vi "Compose email message.vi"(8 "error in (no error)":errorcluster, 11 "DesignRequest":T1={"Project Folder"=path "D:/inetpub/wwwroot/Designs/341406569189", "Method Name"="EtFlocSedFi", "Inputs"=[{"Label.Text"="UI.Name", "Control Type"=4, "Numeric"=0.0, "Array"=[], "status"=FALSE, "Str Array"=[], "String"="Cornell University", "unit"=""}, {"Label.Text"="UI.Email", "Control Type"=4, "Numeric"=0.0, "Array"=[], "status"=FALSE, "Str Array"=[], "String"="mw24@cornell.edu", "unit"=""}, {"Label.Text"="UI.Organization", "Control Type"=4, "Numeric"=0.0, "Array"=[], "status"=FALSE, "Str Array"=[], "String"="Cornell University", "unit"=""}, {"Label.Text"="UI.Language", "Control Type"=4, "Numeric"=0.0, "Array"=[], "status"=FALSE, "Str Array"=[], "String"="English", "unit"=""}, {"Label.Text"="UI.Country", "Control Type"=4, "Numeric"=0.0, "Array"=[], "status"=FALSE, "Str Array"=[], "String"="US", "unit"=""}, {"Label.Text"="UI.ProjectTitle", "Control Type"=4, "Numeric"=0.0, "Array"=[], "status"=FALSE, "Str Array"=[], "String"="testing agian", "unit"=""}, {"Label.Text"="UI.ProjectCity", "Control Type"=4, "Numeric"=0.0, "Array"=[], "status"=FALSE, "Str Array"=[], "String"="Ithaca", "unit"=""}, {"Label.Text"="UI.ProjectState", "Control Type"=4, "Numeric"=0.0, "Array"=[], "status"=FALSE, "Str Array"=[], "String"="New York", "unit"=""}, {"Label.Text"="UI.ProjectNotes", "Control Type"=4, "Numeric"=0.0, "Array"=[], "status"=FALSE, "Str Array"=[], "String"="lots of water", "unit"=""}, {"Label.Text"="Q.Plant", "Control Type"=18, "Numeric"=2145.0, "Array"=[], "status"=FALSE, "Str Array"=[], "String"="", "unit"="L/s"}], "Version"=0}) -> (0 "error out":errorcluster, 3 "DesignRequest out":T1={"Project Folder"=path "D:/inetpub/wwwroot/Designs/341406569189", "Method Name"="EtFlocSedFi", "Inputs"=[{"Label.Text"="UI.Name", "Control Type"=4, "Numeric"=0.0, "Array"=[], "status"=FALSE, "Str Array"=[], "String"="Cornell University", "unit"=""}, {"Label.Text"="UI.Email", "Control Type"=4, "Numeric"=0.0, "Array"=[], "status"=FALSE, "Str Array"=[], "String"="mw24@cornell.edu", "unit"=""}, {"Label.Text"="UI.Organization", "Control Type"=4, "Numeric"=0.0, "Array"=[], "status"=FALSE, "Str Array"=[], "String"="Cornell University", "unit"=""}, {"Label.Text"="UI.Language", "Control Type"=4, "Numeric"=0.0, "Array"=[], "status"=FALSE, "Str Array"=[], "String"="English", "unit"=""}, {"Label.Text"="UI.Country", "Control Type"=4, "Numeric"=0.0, "Array"=[], "status"=FALSE, "Str Array"=[], "String"="US", "unit"=""}, {"Label.Text"="UI.ProjectTitle", "Control Type"=4, "Numeric"=0.0, "Array"=[], "status"=FALSE, "Str Array"=[], "String"="testing agian", "unit"=""}, {"Label.Text"="UI.ProjectCity", "Control Type"=4, "Numeric"=0.0, "Array"=[], "status"=FALSE, "Str Array"=[], "String"="Ithaca", "unit"=""}, {"Label.Text"="UI.ProjectState", "Control Type"=4, "Numeric"=0.0, "Array"=[], "status"=FALSE, "Str Array"=[], "String"="New York", "unit"=""}, {"Label.Text"="UI.ProjectNotes", "Control Type"=4, "Numeric"=0.0, "Array"=[], "status"=FALSE, "Str Array"=[], "String"="lots of water", "unit"=""}, {"Label.Text"="Q.Plant", "Control Type"=18, "Numeric"=2145.0, "Array"=[], "status"=FALSE, "Str Array"=[], "String"="", "unit"="L/s"}], "Version"=0})   [LabVIEW 2012, in "Design Server.lvlib"]
uses:
  Design Server.lvlib
  Design Request.ctl
  Variable cluster.ctl
  RequestKeys.ctl
  ReadWrite.ctl
  ADT 2/AguaClara Library.lvlib
panel:
  out "Project URL":string
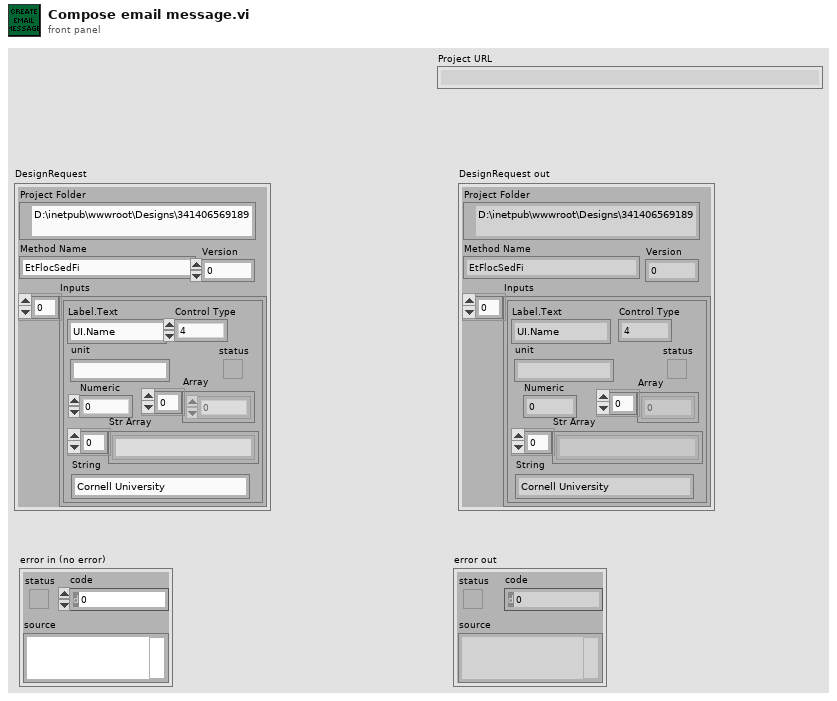
[diagram p1: front panel]
types:
  T1 = typedef "Design Server.lvlib/Design Request.ctl" = cluster{"Project Folder":path, "Method Name":string, "Inputs":T2, "Version":i32}
  T2 = typedef "Design Server.lvlib/Variable cluster.ctl" = cluster{"Label.Text":string, "Control Type":u32, "Numeric":dbl, "Array":dbl[], "status":bool, "Str Array":string[], "String":string, "unit":string}[]
  T3 = typedef "Design Server.lvlib/RequestKeys.ctl" = enum16{"FormName", "Name", "Email", "Organization", "Country", "ProjectTitle", "ProjectCity", "ProjectState", "ProjectNotes"}
  T4 = typedef "ReadWrite.ctl" = enum16{"Read", "Write"}
  T5 = typedef "Mail Server.ctl" = cluster{"Outgoing Mail Server (SMTP)":string, "MAIL Account User ID":string, "MAIL Account Password":string, "Enable SSL":bool, "Port":i32, "Sender's Email Address":string, "Sender's Name":string}
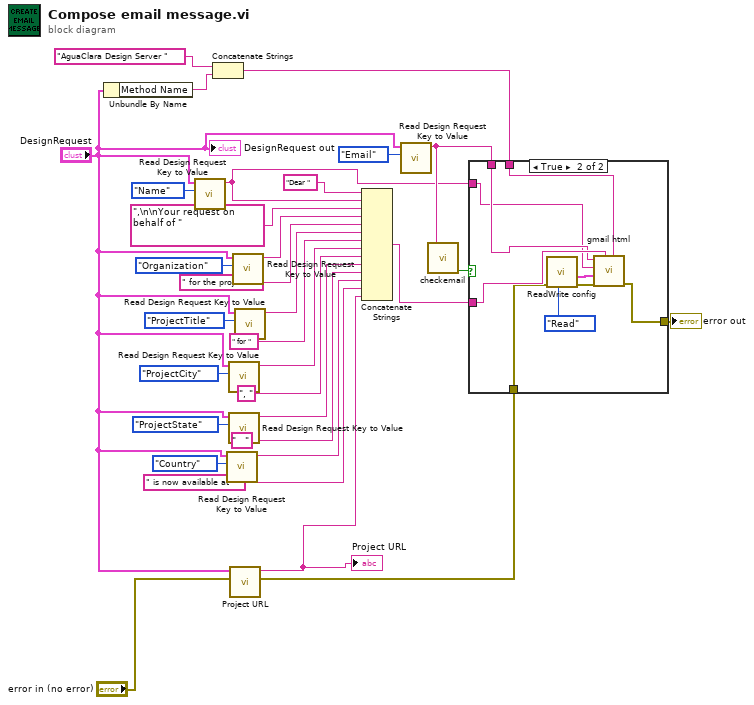
[diagram p0: block diagram]
diagram:
  n1 = Unbundle By Name("DesignRequest") -> ("Method Name"=w8:string)
  n2 = call "Read Design Request Key to Value.vi"("Request Keys"=RequestKeys."Name", "DesignRequest"="DesignRequest") -> ("Value"=w1:string)  [unwired: 9 in]
  n3 = Concatenate Strings("AguaClara Design Server " ("subject ([No Subject])"), w8) -> (w7:string)
  n4 = call "Read Design Request Key to Value.vi"("Request Keys"=RequestKeys."Country", "DesignRequest"="DesignRequest") -> ("Value"=w18:string)  [unwired: 9 in]
  n5 = call "Read Design Request Key to Value.vi"("Request Keys"=RequestKeys."ProjectCity", "DesignRequest"="DesignRequest") -> ("Value"=w24:string)  [unwired: 9 in]
  n6 = call "Read Design Request Key to Value.vi"("Request Keys"=RequestKeys."ProjectState", "DesignRequest"="DesignRequest") -> ("Value"=w20:string)  [unwired: 9 in]
  n7 = call "Project URL.vi"("error in (no error)"="error in (no error)", "DesignRequest"="DesignRequest") -> ("error out"=w4:errorcluster, "Project URL"=w5:string)  [unwired: 8 in]
  "Project URL" <- w5
  n8 = call "Read Design Request Key to Value.vi"("Request Keys"=RequestKeys."Organization", "DesignRequest"="DesignRequest") -> ("Value"=w27:string)  [unwired: 9 in]
  n9 = call "Read Design Request Key to Value.vi"("Request Keys"=RequestKeys."ProjectTitle", "DesignRequest"="DesignRequest") -> ("Value"=w16:string)  [unwired: 9 in]
  n10 = Concatenate Strings("Dear ", w1, ",\n\nYour request on behalf of " ("string"), w27, " for the project " ("string"), w16, " for " ("string"), w24, ", " ("string"), w20, "   " ("string"), w18, " is now available at " ("string"), w5) -> (w12:string)
  n11 = call "Read Design Request Key to Value.vi"("Request Keys"=RequestKeys."Email", "DesignRequest"="DesignRequest") -> ("Value"=w3:string)  [unwired: 9 in]
  n12 = call "checkemail.vi"("email"=w3) -> ("valid email"=w2:bool)  [unwired: 7 in, 3 out]
  n13 = case shown="True" w2 {
    tunnel: w12 -> [_ w38]
    tunnel: [w32 w34] -> w11
    tunnel: w7 -> [_ w39]
    tunnel: w4 -> [w32 w33]
    tunnel: w3 -> [_ w37]
    tunnel: w1 -> [_ w36]
    frame False {
    }
    frame True {
      n14 = call "ReadWrite config.vi"("Config"=ReadWrite."Read", "error in (no error)"=w33) -> ("error out"=w35:errorcluster, "Mail Server"=w41:T5)  [unwired: 6 in, 2 out]
      n15 = call "gmail html.vi"("Subject"=w39, "Body"=w38, "error in (no error)"=w35, "Server"=w41, "Recipient's Name"=w36, "Recipient's Email Address"=w37) -> ("error out"=w34:errorcluster)  [unwired: 5 in]
    }
  }
  "error out" <- w11
  "DesignRequest out" <- "DesignRequest"
